vi "Time2Unix_time.vi"() -> (2 "seconds since 1Jan1904":timestamp, 3 "Numerisch":dbl)   [LabVIEW 2013]
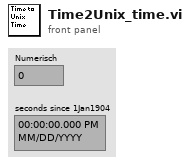
[diagram p1: front panel]
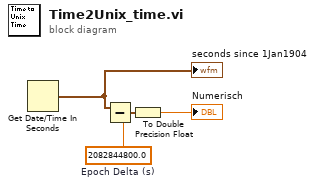
[diagram p0: block diagram]
diagram:
  w4 = 2082844800.0  # Epoch Delta (s)
  n1 = Get Date/Time In Seconds() -> (seconds since 1Jan1904=w2:timestamp)
  "seconds since 1Jan1904" <- w2
  n2 = Subtract(x=w2, y=w4) -> (x-y=w1:timestamp)
  n3 = To Double Precision Float(number=w1) -> (double precision float=→"Numerisch":dbl)
